vi "Image Processing SubVI.vi"(8 "Error In":errorcluster, 11 "Image Refnum In":T2) -> (0 "Error Out":errorcluster, 2 "Shape Report":T1(array[cluster]) {"Score" format="%.2f"; "Centroid"."y" format="%.2f"; "Centroid"."x" format="%.2f"}, 3 "Image Refnum Out":T2)   [LabVIEW 2014]
doc: "This subVI takes in an image and performs some image processing. The algorithm used outputs a shape report of a licence plate, and also outputs the image as a binary which has been condensed to near enough just the license plate alphanumeric numbers."
uses:
  <vilib>/vision/Image Controls.llb/IMAQ Image.ctl
  <vilib>/vision/NI_Vision_Development_Module.lvlib
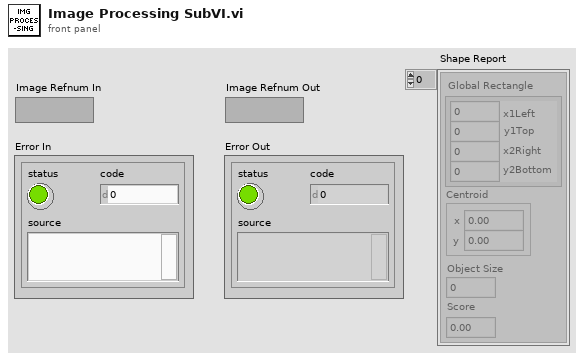
[diagram p1: front panel]
types:
  T1 = cluster{"Global Rectangle":cluster{"x1Left":i32, "y1Top":i32, "x2Right":i32, "y2Bottom":i32}, "Centroid":cluster{"x":sgl, "y":sgl}, "Object Size":u32, "Score":dbl}[]
  T2 = typedef "IMAQ Image.ctl" = refnum<image>
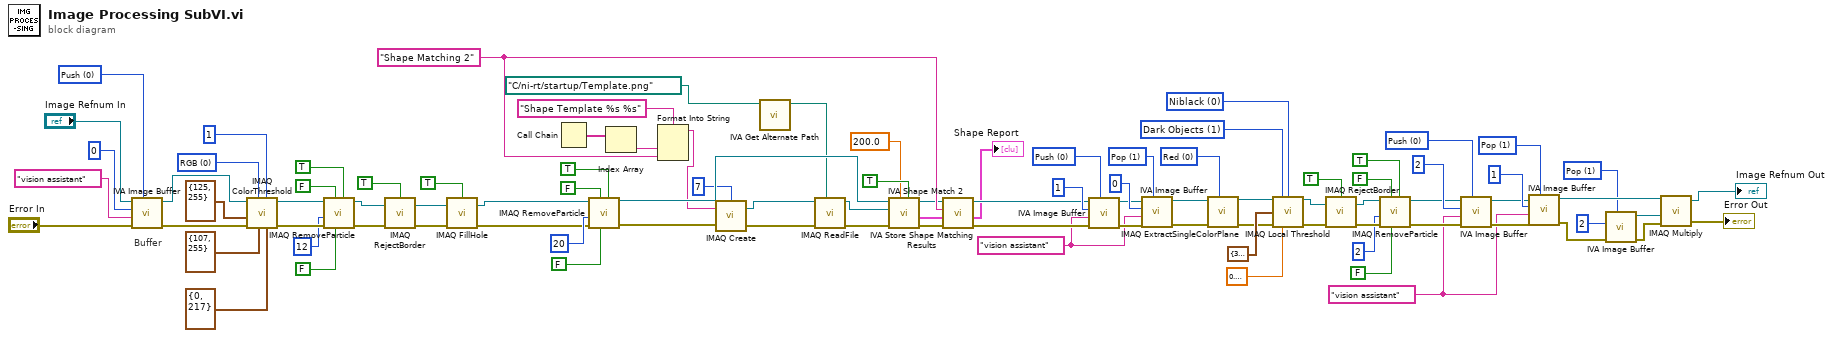
[diagram p0: block diagram]
diagram:
  w87 = u16 1 items=["Push", "Pop", "Reset"] ("Function")
  w85 = u16 1 items=["Push", "Pop", "Reset"] ("Function")
  w13 = "vision assistant" ("Prefix")
  w81 = u16 0 items=["Push", "Pop", "Reset"] ("Function")
  w69 = u32 1 items=["Bright Objects", "Dark Objects"] ("Look For (Bright Objects)")
  w66 = u32 0 items=["Niblack", "Background Correction"] ("Method")
  w61 = 0 items=["Red", "Green", "Blue", "Hue", "Saturation", "Luminance", "Value", "Intensity"] ("Color Plane")
  w59 = u16 1 items=["Push", "Pop", "Reset"] ("Function")
  w14 = "vision assistant" ("Prefix")
  w55 = u16 0 items=["Push", "Pop", "Reset"] ("Function")
  w52 = "Shape Matching 2" ("Step Name")
  w21 = u16 0 items=["RGB", "HSL", "HSV", "HSI"] ("Color Mode")
  w17 = u16 0 items=["Push", "Pop", "Reset"] ("Function")
  # "Buffer"
  n1 = call <vilib>:"IVA Image Buffer.vi"("Function"=w17, "error in (no error)"="Error In", "Prefix"="vision assistant", "Buffer #"=0, "Image In"="Image Refnum In") -> ("error out"=w26:errorcluster, "Image Out"=w25:T2)  [unwired: 5 out]
  n2 = call "IMAQ ColorThreshold"("Blue or Luma or Val or Inten Range"=cluster{"Lower value":i32, "Upper value":i32} {"Lower value"=0, "Upper value"=217}, "Replace Value"=1, "Green or Sat Range"=cluster{"Lower value":i32, "Upper value":i32} {"Lower value"=107, "Upper value"=255}, "Color Mode"=w21, "error in (no error)"=w26, "Red or Hue Range"=cluster{"Lower value":i32, "Upper value":i32} {"Lower value"=125, "Upper value"=255}, "Image Src"=w25) -> ("error out"=w32:errorcluster, "Image Dst Out"=w31:T2)  [unwired: 1 in, 2 out]
  n3 = call "IMAQ RemoveParticle"("Connectivity 4/8 (8)"=TRUE, "Low Pass/High Pass (Low)"=FALSE, "Square/Hexa (Square)"=FALSE, "error in (no error)"=w32, "Number of Erosion"=12, "Image Src"=w31) -> ("error out"=w35:errorcluster, "Image Dst Out"=w34:T2)  [unwired: 1 in, 3 out]
  n4 = call "IMAQ RejectBorder"("error in (no error)"=w35, "Image Src"=w34, "Connectivity 4/8 (8)"=TRUE) -> ("error out"=w38:errorcluster, "Image Dst Out"=w37:T2)  [unwired: 1 in, 2 out]
  n5 = call "IMAQ FillHole"("error in (no error)"=w38, "Image Src"=w37, "Connectivity 4/8 (8)"=TRUE) -> ("error out"=w3:errorcluster, "Image Dst Out"=w4:T2)  [unwired: 1 in, 2 out]
  n6 = Call Chain() -> (call chain=w8:string[])
  n7 = call "IMAQ RemoveParticle"("Connectivity 4/8 (8)"=TRUE, "Low Pass/High Pass (Low)"=FALSE, "Square/Hexa (Square)"=FALSE, "error in (no error)"=w3, "Number of Erosion"=20, "Image Src"=w4) -> ("error out"=w5:errorcluster, "Image Dst Out"=w45:T2)  [unwired: 1 in, 3 out]
  n8 = Index Array(array=w8) -> (element=w7:string)  [unwired: 1 in]
  n9 = Format Into String(format string="Shape Template %s %s" ("Image Name"), w7, w52) -> (resulting string=w11:string)  [unwired: 2 in, 1 out]
  n10 = call "IMAQ Create"("Border Size"=7, "Image Name"=w11, "error in (no error)"=w5) -> ("New Image"=w2:T2, "error out"=w1:errorcluster)  [unwired: 1 in, 1 out]
  n11 = call <vilib>:"IVA Get Alternate Path.vi"("Path In"=path "C:/ni-rt/startup/Template.png" ("Template Path")) -> ("Path Out"=w6:path)  [unwired: 10 out]
  n12 = call "IMAQ ReadFile"("File Path"=w6, "error in (no error)"=w1, "Image"=w2) -> ("error out"=w50:errorcluster, "Image Out"=w51:T2)  [unwired: 2 in, 5 out]
  n13 = call <vilib>:"IVA Shape Match 2.vi"("Scale Invariance"=TRUE, "Minimal Score"=200.0, "error in (no error)"=w50, "Template"=w51, "Image Src"=w45) -> ("error out"=w46:errorcluster, "Shape Report"=w47:T1, "Image Out"=w48:T2)  [unwired: 4 out]
  n14 = call <vilib>:"IVA Store Shape Matching Results.vi"("error in (no error)"=w46, "Shape Report"=w47, "Step Name"=w52, "Image in"=w48) -> ("error out"=w54:errorcluster, "Shape Report (calibrated)"=→"Shape Report":T1, "Image dup"=w53:T2)  [unwired: 5 out]
  n15 = call <vilib>:"IVA Image Buffer.vi"("Function"=w55, "error in (no error)"=w54, "Prefix"=w14, "Buffer #"=1, "Image In"=w53) -> ("error out"=w58:errorcluster, "Image Out"=w57:T2)  [unwired: 5 out]
  n16 = call <vilib>:"IVA Image Buffer.vi"("Function"=w59, "error in (no error)"=w58, "Prefix"=w14, "Buffer #"=0, "Image In"=w57) -> ("error out"=w63:errorcluster, "Image Out"=w62:T2)  [unwired: 5 out]
  n17 = call "IMAQ ExtractSingleColorPlane"("Color Plane"=w61, "error in (no error)"=w63, "Image Src"=w62) -> ("error out"=w64:errorcluster, "Image Dst Out"=w65:T2)  [unwired: 1 in, 6 out]
  n18 = call "IMAQ Local Threshold"("Image Src"=w65, "Look For (Bright Objects)"=w69, "Method (Niblack)"=w66, "Window Size (32x32)"=cluster{"SizeX":i32, "SizeY":i32} {"SizeX"=32, "SizeY"=32} ("Kernel Size"), "error in (no error)"=w64, "Niblack Deviation Factor (0.2)"=0.20000000000000004 ("Niblack Deviation Factor")) -> ("Image Dst Out"=w71:T2, "error out"=w72:errorcluster)  [unwired: 2 in, 6 out]
  n19 = call "IMAQ RejectBorder"("error in (no error)"=w72, "Image Src"=w71, "Connectivity 4/8 (8)"=TRUE) -> ("error out"=w78:errorcluster, "Image Dst Out"=w77:T2)  [unwired: 1 in, 2 out]
  n20 = call "IMAQ RemoveParticle"("Connectivity 4/8 (8)"=TRUE, "Low Pass/High Pass (Low)"=FALSE, "Square/Hexa (Square)"=FALSE, "error in (no error)"=w78, "Number of Erosion"=2, "Image Src"=w77) -> ("error out"=w80:errorcluster, "Image Dst Out"=w79:T2)  [unwired: 1 in, 3 out]
  n21 = call <vilib>:"IVA Image Buffer.vi"("Function"=w81, "error in (no error)"=w80, "Prefix"=w13, "Buffer #"=2, "Image In"=w79) -> ("error out"=w84:errorcluster, "Image Out"=w83:T2)  [unwired: 5 out]
  n22 = call <vilib>:"IVA Image Buffer.vi"("Function"=w85, "error in (no error)"=w84, "Prefix"=w13, "Buffer #"=1, "Image In"=w83) -> ("error out"=w92:errorcluster, "Image Out"=w91:T2)  [unwired: 5 out]
  n23 = call <vilib>:"IVA Image Buffer.vi"("Function"=w87, "error in (no error)"=w92, "Buffer #"=2) -> ("error out"=w90:errorcluster, "Image Out"=w89:T2)  [unwired: 2 in, 5 out]
  n24 = call "IMAQ Multiply"("Image Src A"=w91, "Image Src B"=w89, "error in (no error)"=w90) -> ("Image Dst Out"=→"Image Refnum Out":T2, "error out"=→"Error Out":errorcluster)  [unwired: 2 in, 2 out]
